vi "Magazine_Globals.vi"() -> ()   [LabVIEW 2019]
uses:
  Subsystems/Magazine/Magazine_Cluster.ctl
panel:
  in  "Magazine_Execute_Notifier":refnum<notifier>
  in  "Magazine_Set_Notifier":refnum<notifier>
  in  "Magazine_Execute_Ref":string
  in  "Magazine_Set_Ref":string
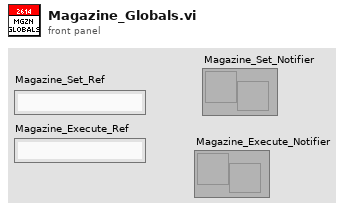
[diagram p1: front panel]
diagram:
